vi "Configure Acquisition.vi"(8 "error in (no error)":errorcluster, 11 "Fetch Waveforms CFG in":refnum<class "Fetch Waveforms CFG.lvclass">) -> (0 "error out":errorcluster, 3 "Fetch Waveforms CFG out":refnum<class "Fetch Waveforms CFG.lvclass">)   [LabVIEW 2023, in "PXIe-4353.lvlib" / "Fetch Waveforms CFG.lvclass"]
uses:
  Fetch Waveforms CFG.lvclass
  D:/git/HAL/Configuration Base/Configuration Base.lvclass
  Configuration Base/Configuration Base.lvclass/Configuration Base.ctl
  Fetch Waveforms CFG.lvclass/Fetch Waveforms CFG.ctl
  d4a19599-12e2-4694-835e-9d65542d9fb2.vi
  5c8cdaef-3b3b-48b1-a5b4-8435a3432539.vi
  <vilib>/JDP Science/JSONtext/Next JSON Value.vi
  <vilib>/JDP Science/JSONtext/String Subset.vi
  <vilib>/JDP Science/JSONtext/Parsing/Advance past next JSON Value (inlined COPY).vi
  <vilib>/JDP Science/JSONtext/Parsing/Advance past whitespace.vi
  <vilib>/JDP Science/JSONtext/Parsing/Advance past String.vi
  <vilib>/JDP Science/JSONtext/Parsing/Advance past Number.vi
  <vilib>/JDP Science/JSONtext/Parsing/Advance past Line Ending.vi
  <vilib>/JDP Science/JSONtext/Parsing/Parse Full Path or Item Name.vi
  <vilib>/JDP Science/JSONtext/Parsing/Advance past Array.vi
  <vilib>/JDP Science/JSONtext/Parsing/Advance past Object.vi
  <vilib>/JDP Science/JSONtext/support/Error Cluster From Code.vi
  <vilib>/JDP Science/JSONtext/Offset/Find Item Locations by Path.vi
  <vilib>/JDP Science/JSONtext/JSON text to Variant.vi
  <vilib>/Utility/error.llb/Error Cluster From Error Code.vi
  <vilib>/JDP Science/JSONtext/LVClass Serializer/JSONtext LVClass Serializer.lvclass
  <vilib>/ErrorRing/Error Ring.xnode
  Configuration Base/Configuration Base.lvclass
  <vilib>/JDP Science/JSONtext/JSONtext.lvlib
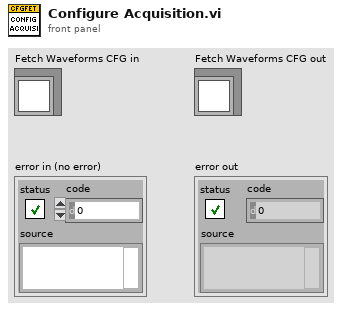
[diagram p1: front panel]
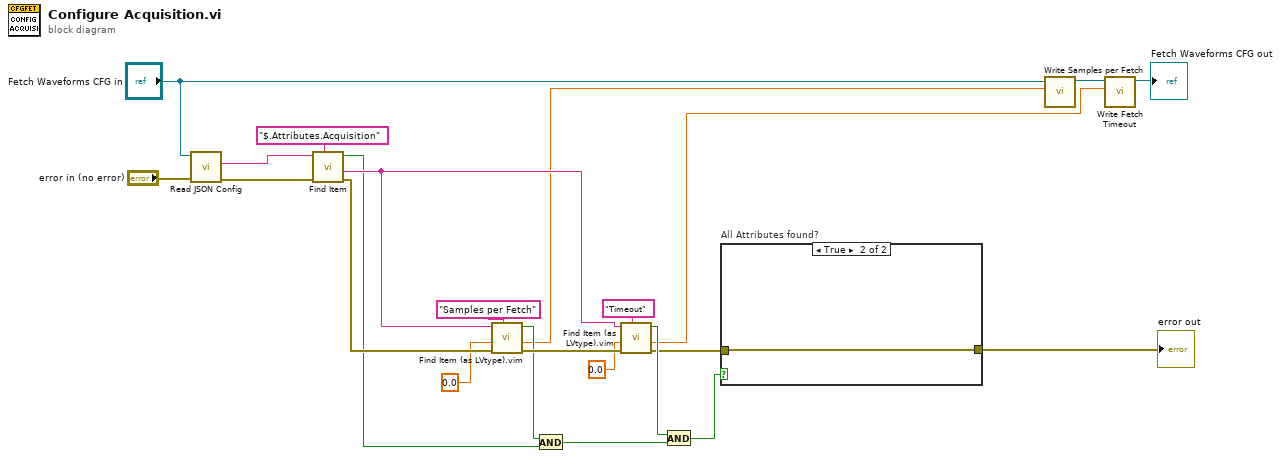
[diagram p0: block diagram]
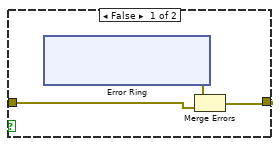
[diagram p2: hidden frame]
diagram:
  n1 = call "Read JSON Config.vi"("error in"="error in (no error)", "object in"="Fetch Waveforms CFG in") -> ("error out"=w23:errorcluster, "<JSON>Config"=w22:string)  [unwired: 7 in, 1 out]
  n2 = call <vilib>:"Find Item.vi"("$Path or Item Name"="$.Attributes.Acquisition", "error in (no error)"=w23, "JSON"=w22) -> ("error out"=w21:errorcluster, "<JSON>"=w19:string, "Found"=w11:bool)  [unwired: 5 in, 1 out]
  n3 = call "Find Item (as LVtype).vim"("$Path or Item Name"="Samples per Fetch", "error in (no error)"=w21, "Data Type and Default Value"=0.0, "JSON"=w19) -> ("error out"=w17:errorcluster, "Data"=w4:dbl, "Found"=w15:bool)  [unwired: 4 in, 1 out]
  n4 = And(x=w15, y=w11) -> (x .and. y?=w13:bool)
  n5 = call "Find Item (as LVtype).vim"("$Path or Item Name"="Timeout", "error in (no error)"=w17, "Data Type and Default Value"=0.0, "JSON"=w19) -> ("error out"=w7:errorcluster, "Data"=w3:dbl, "Found"=w14:bool)  [unwired: 4 in, 1 out]
  n6 = And(x=w14, y=w13) -> (x .and. y?=w2:bool)
  n7 = case "All Attributes found?" shown="True" w2 {
    tunnel: w7 -> [w24 w32]
    tunnel: [w25 w32] -> w6
    frame False {
      n8 = xnode "Error Ring"() -> ("error out"=w26:errorcluster)
      n9 = Merge Errors(w26, w24) -> (w25:errorcluster)
    }
    frame True {
    }
  }
  "error out" <- w6
  n10 = call "Write Samples per Fetch.vi"("Samples per Loop"=w4, "Fetch Waveforms CFG in"="Fetch Waveforms CFG in") -> ("Fetch Waveforms CFG out"=w9:refnum<class "Fetch Waveforms CFG.lvclass">)  [unwired: 8 in, 1 out]
  n11 = call "Write Fetch Timeout.vi"("Fetch Timeout"=w3, "Fetch Waveforms CFG in"=w9) -> ("Fetch Waveforms CFG out"=→"Fetch Waveforms CFG out":refnum<class "Fetch Waveforms CFG.lvclass">)  [unwired: 8 in, 1 out]
